vi "LaguerreGaussLUTGenerator.vi"(1 "beam waist w0 (in m; default 1E-4 = 0.1mm)":dbl, 2 "l":i16, 3 "p":i16, 4 "beam parameters":T1={"amplitudeMatrix"=[], "SLM width (m)"=0.01498, "SLM height (m)"=0.01092, "wavelength (m)"=6.33e-07, "Resolution x"=1920, "Resolution y"=1080} caption="Beam Parameters, dependant on SLM and LASER" {"Resolution x" format="%#.0f"; "SLM width (m)" format="%_6f"; "SLM height (m)" format="%#_6f"}) -> (0 "Look-up Table":T2)   [LabVIEW 2024]
uses:
  typeDefs/BPandSLM.ctl
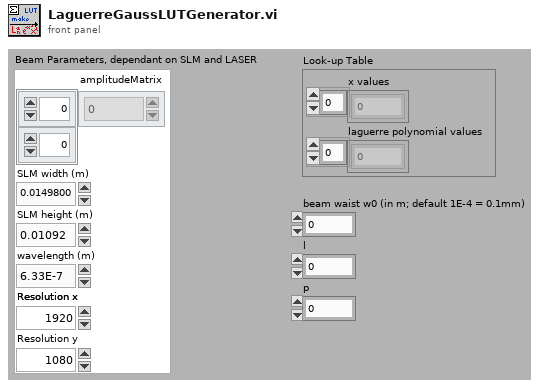
[diagram p1: front panel]
types:
  T1 = typedef "BPandSLM.ctl" = cluster{"amplitudeMatrix":csg[][], "SLM width (m)":dbl, "SLM height (m)":dbl, "wavelength (m)":dbl, "Resolution x":u32, "Resolution y":u32}
  T2 = cluster{"x values":dbl[], "laguerre polynomial values":dbl[]}
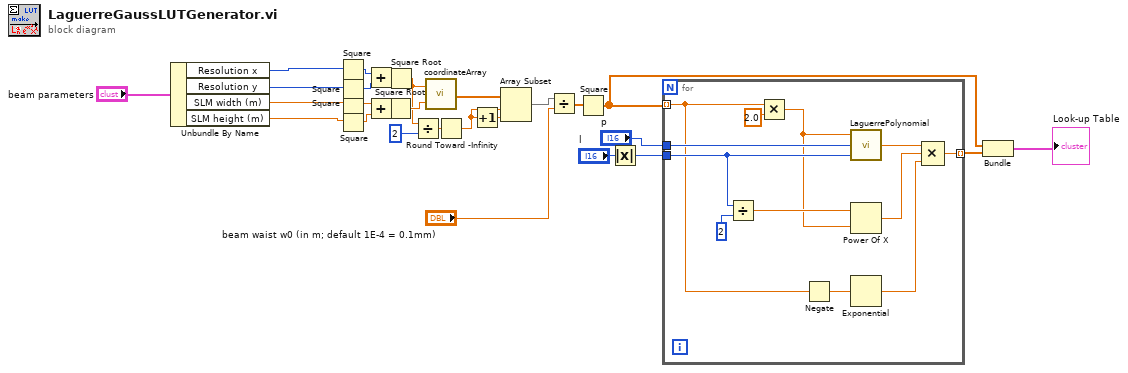
[diagram p0: block diagram]
diagram:
  n1 = Unbundle By Name("beam parameters") -> ("Resolution x"=w6:u32, "Resolution y"=w9:u32, "SLM width (m)"=w8:dbl, "SLM height (m)"=w7:dbl)
  n2 = Square(x=w6) -> (x^2=w10:u32)
  n3 = Square(x=w9) -> (x^2=w11:u32)
  n4 = Square(x=w8) -> (x^2=w12:dbl)
  n5 = Square(x=w7) -> (x^2=w13:dbl)
  n6 = Add(x=w10, y=w11) -> (x+y=w15:u32)
  n7 = Add(x=w12, y=w13) -> (x+y=w14:dbl)
  n8 = Square Root(x=w14) -> (sqrt(x)=w26:dbl)
  n9 = Square Root(x=w15) -> (sqrt(x)=w25:dbl)
  n10 = Divide(x=w25, y=2) -> (x/y=w18:dbl)
  n11 = call "coordinateArray.vi"("width of represented x (or y) range (in m; default 1E-3=1mm)"=w26, "array size (default 64)"=w25) -> ("x array"=w17:sgl[])
  n12 = Round Toward -Infinity(1:w18) -> (0:w19:dbl)
  n13 = Increment(x=w19) -> (x+1=w20:dbl)
  n14 = Array Subset(array=w17, index=w19, length=w20) -> (w23:sgl[])
  n15 = Divide(x=w23, y="beam waist w0 (in m; default 1E-4 = 0.1mm)") -> (x/y=w22:dbl[])
  n16 = Square(x=w22) -> (x^2=w2:dbl[])
  n17 = Absolute Value(x="l") -> (abs(x)=w3:i16)
  n18 = for {
    tunnel: w3 -> [w35]
    tunnel: "p" -> [w39]
    tunnel: w2 -> [w32] mode=indexing
    tunnel: [w31] -> w21 mode=indexing
    n19 = Divide(x=w35, y=i16 2) -> (x/y=w36:dbl)
    n20 = Multiply(x=w32, y=2.0) -> (x*y=w34:dbl)
    n21 = Negate(x=w32) -> (-x=w33:dbl)
    n22 = call "LaguerrePolynomial.vi"("a"=w35, "n"=w39, "x"=w34) -> ("associated Laguerre polynomial (n,a,x)"=w30:dbl)
    n23 = Power Of X(1:w34, 2:w36) -> (0:w29:dbl)
    n24 = Exponential(1:w33) -> (0:w28:dbl)
    n25 = Compound Arithmetic op=MULTIPLY(w30, w29, w28) -> (w31:dbl)
  }
  n26 = Bundle(w2, w21) -> (→"Look-up Table":cluster{dbl[], dbl[]})  [unwired: 1 in]
